vi "Configure Secured Parameter Protection.vi"(8 "error in (no error)":errorcluster, 9 "enable protection":bool, 10 "node address (same)":u8, 11 "ProPar in":refnum<class "PL Bronkhorst ProPar.lvclass">) -> (0 "error out":errorcluster, 3 "ProPar out":refnum<class "PL Bronkhorst ProPar.lvclass">)   [LabVIEW 2015, in "PL Bronkhorst ProPar.lvclass"]
doc: "Enables secured parameter changing of the specified <b>node</b>."
uses:
  PL Bronkhorst ProPar.lvclass
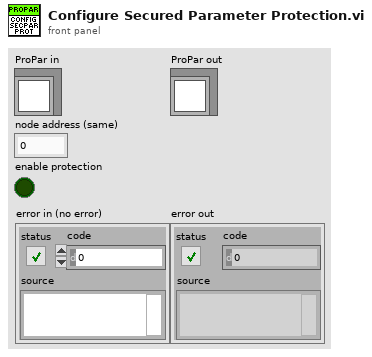
[diagram p1: front panel]
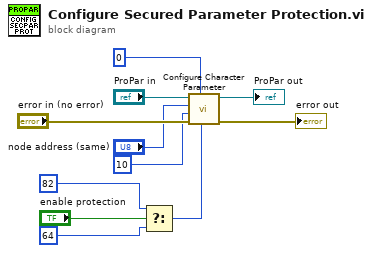
[diagram p0: block diagram]
diagram:
  n1 = Select(t=u8 82 ("value"), s="enable protection", f=u8 64 ("value")) -> (s? t:f=w1:u8)
  n2 = call "Configure Character Parameter.vi"("value"=w1, "process number"=u8 0, "error in (no error)"="error in (no error)", "parameter number"=u8 10 ("process number"), "node"="node address (same)", "ProPar in"="ProPar in") -> ("error out"=→"error out":errorcluster, "ProPar out"=→"ProPar out":refnum<class "PL Bronkhorst ProPar.lvclass">)  [unwired: 4 in]
